vi "Xeryon Axis driver.vi"(4 "Config":T1, 5 "Stage index":u32) -> ()   [LabVIEW 2014]
uses:
  <vilib>/Utility/error.llb/DialogType.ctl
  Serial driver/Serial parameters.ctl
  Xeryon Axis command.ctl
  Xeryon status bits.ctl
  Axis Manager/Axis config.ctl
  Axis Manager/Axis enum.ctl
panel:
  out "Latched setpoint":dbl
  in  "Save":bool
  in  "Recover":bool
  in  "Reset encoder":bool
  in  "Apply settings file":bool
  in  "Settings file":path
  in  "Tab Control":enum32{"Status", "Graphs", "Feedback"}(tab)
  out "Within Tolerance":bool
  out "Statusbits":T3
  out "Actual position":dbl
  out "Serial number":i32
  out "Software number":i32
  out "Stage type":string
  out "Waveform Chart":T4(graph)
  out "Multicolumn Listbox":i32(listbox)
  in  "Continue":bool
  in  "Stop":bool
  in  "Go":bool
  in  "Desired speed":dbl=10.0
  in  "Desired position":dbl
  in  "Step size":dbl=1.0
  in  "Step +X":bool
  in  "Step -X":bool
  in  "Scan +X":bool
  in  "Scan -X":bool
  in  "Find index":bool
  in  "Reset":bool
  out "History :":i32(listbox)=-1
  out "Send feedback":bool
  # "Controls"
  # "In working units (°/mm)"
  # "In working units (°/mm)"
  # "Rotation :  deg/s  - Linear : mm/s"
  # "In working units"
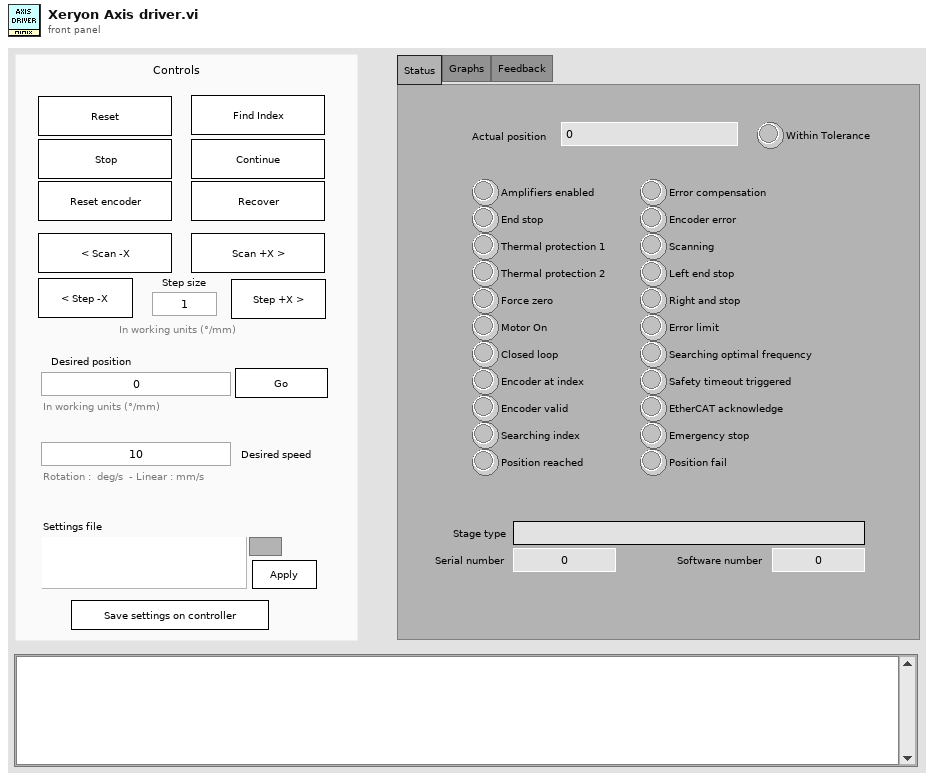
[diagram p1: front panel]
types:
  T1 = typedef "Axis config.ctl" = cluster{"Letter":string, "Stagetype":T2}
  T2 = typedef "Axis enum.ctl" = enum16{"XLA with 50 µm resolution", "XLA with 10 µm resolution", "XLA with 1250 nm resolution", "XLA with 312 nm resolution", "XLA with 78 nm resolution", "XLS with 1250 nm resolution", "XLS with 312 nm resolution", "XLS with 78nm resolution", "XLS with 5nm resolution", "XLS with 1 nm resolution", "XRT-A with 109 µrad resolution", "XRT-U-30 with 109 µrad resolution", "XRT-U-30 with 49 µrad resolution", "XRT-U-30 with 19 µrad resolution", "XRT-U-30 with 3 µrad resolution", "XRT-U-40 with 109 µrad resolution", "XRT-U 40 with 49 µrad resolution", "XRT-U-40 with 19 µrad resolution", "XRT-U-40 with 3 µrad resolution", "XRT-U-60 with 109 µrad resolution", "XRT-U-60 with 49 µrad resolution", "XRT-U-60 with 19 µrad resolution", "XRT-U-60 with 3 µrad resolution"}
  T3 = typedef "Xeryon status bits.ctl" = cluster{"Amplifiers enabled":bool, "End stop":bool, "Thermal protection 1":bool, "Thermal protection 2":bool, "Force zero":bool, "Motor On":bool, "Closed loop":bool, "Encoder at index":bool, "Encoder valid":bool, "Searching index":bool, "Position reached":bool, "Error compensation":bool, "Encoder error":bool, "Scanning":bool, "Left end stop":bool, "Right and stop":bool, "Error limit":bool, "Searching optimal frequency":bool, "Safety timeout triggered":bool, "EtherCAT acknowledge":bool, "Emergency stop":bool, "Position fail":bool}
  T4 = cluster{"Value out":dbl, "Latched setpoint":dbl, i16}
  T5 = enum16{"Position : From user units", "Position : To user units"}
  T6 = typedef "Xeryon Axis command.ctl" = cluster{"Command":enum16{"Reset", "Zero output", "Go home", "Find index", "Scan -X", "Scan +X", "Scan Stop", "Step -X", "Step +X", "Set DPOS", "Stop", "Continue", "Desired speed", "Apply settings file", "Exit", "Reset encoder", "Recover", "Save"}, "Data to send":string}
  T7 = enum16{"Init", "Set stage data", "Update position", "Get"}
  T8 = typedef "Serial parameters.ctl" = enum16{"Serial number", "Software number", "Type of stage", "Status", "Frequency", "Encoder position", "Desired position", "Info", "Phase correction", "Timestamp", "Proportional control factor", "Sync", "XRT1", "XRT3", "XRTA", "XLS1", "XLS3", "XLA1", "XLA3"}
  T9 = enum16{"Reset", "Zero output", "Go home", "Find index", "Scan -X", "Scan +X", "Scan Stop", "Step -X", "Step +X", "Set DPOS", "Stop", "Continue", "Desired speed", "Apply settings file", "Exit", "Reset encoder", "Recover", "Save"}
  T10 = cluster{"Parameters out":T8[], "Values out":i32[], "Stage type":string, "Stage letter":string}
  T11 = typedef "DialogType.ctl" = u16
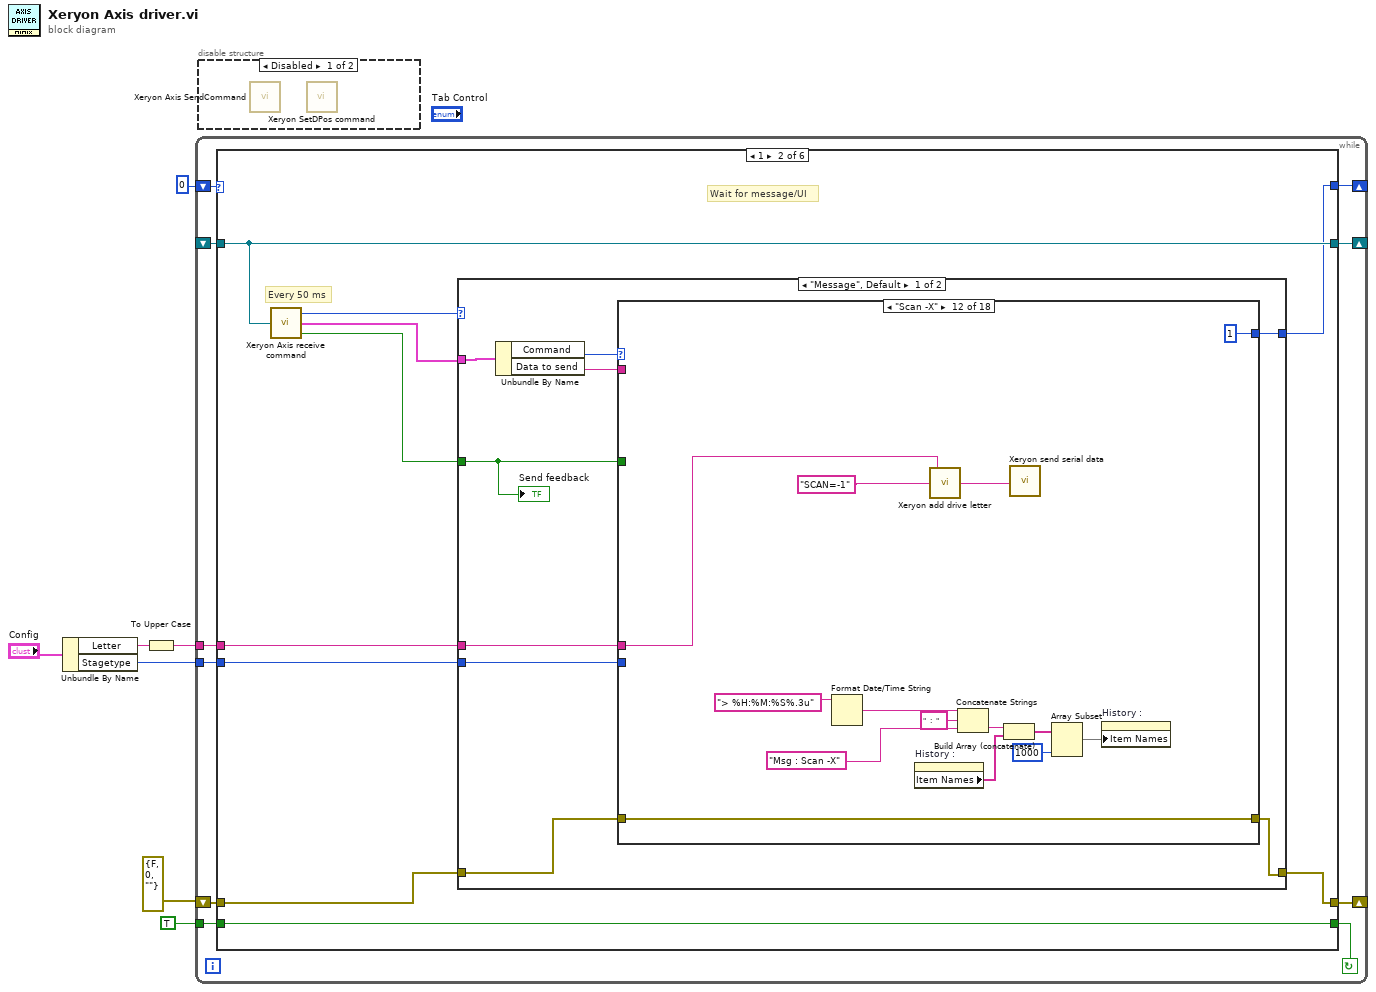
[diagram p0: block diagram]
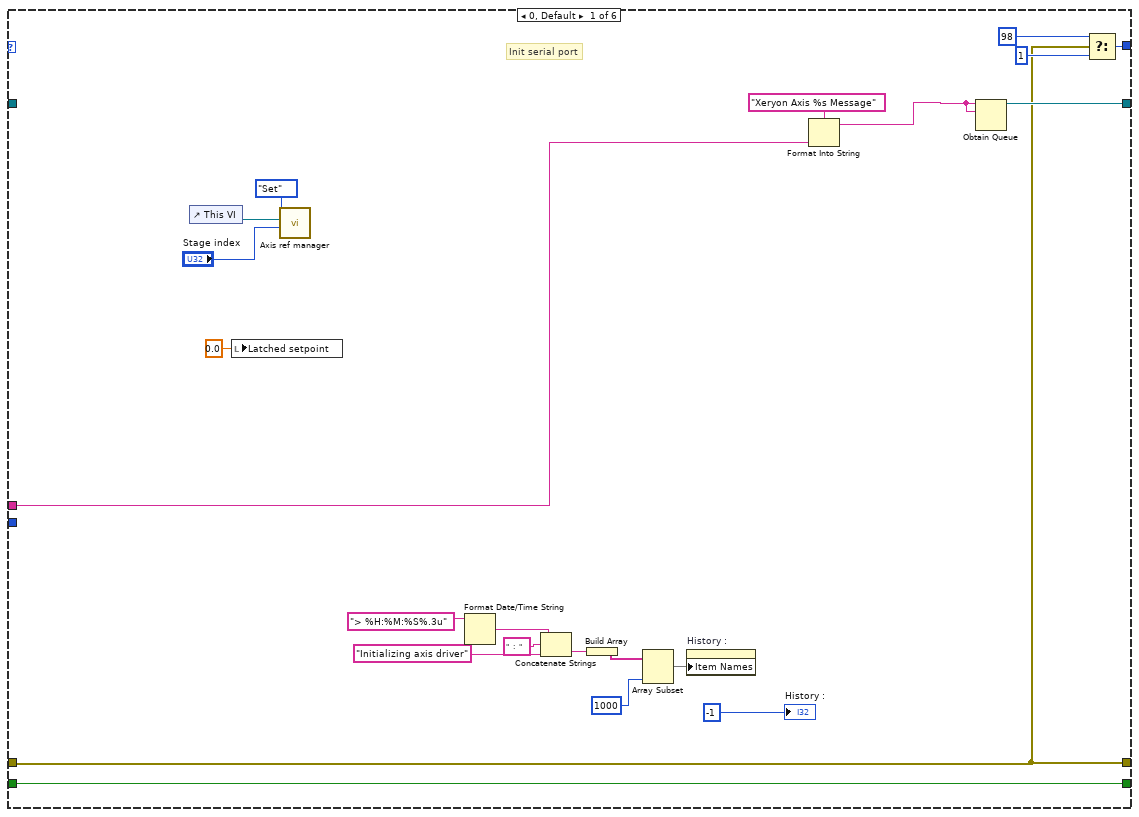
[diagram p3: hidden frame]
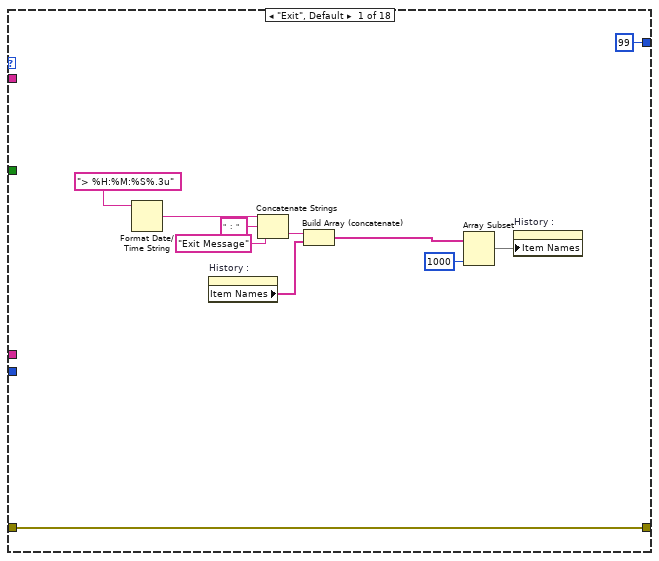
[diagram p4: hidden frame]
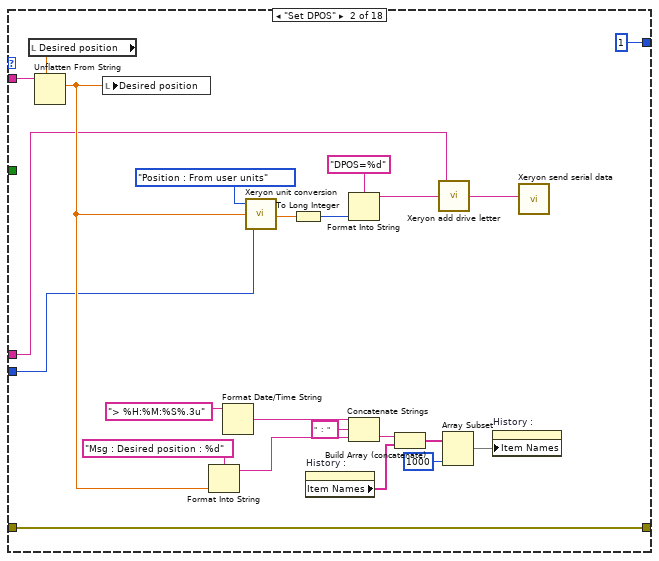
[diagram p5: hidden frame]
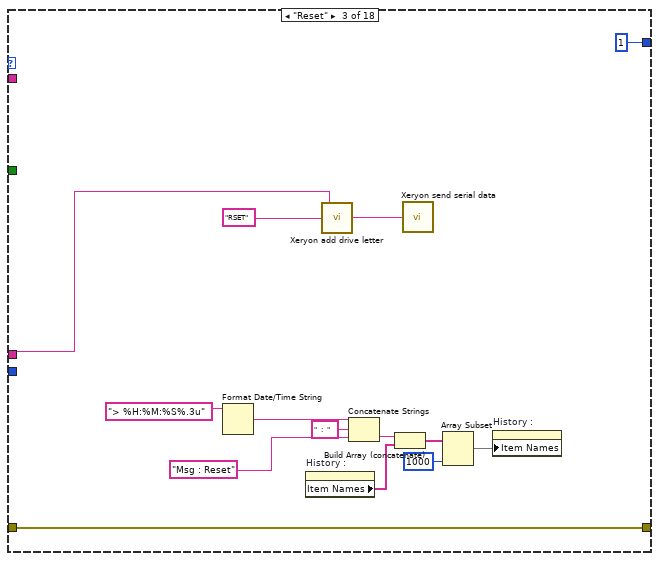
[diagram p6: hidden frame]
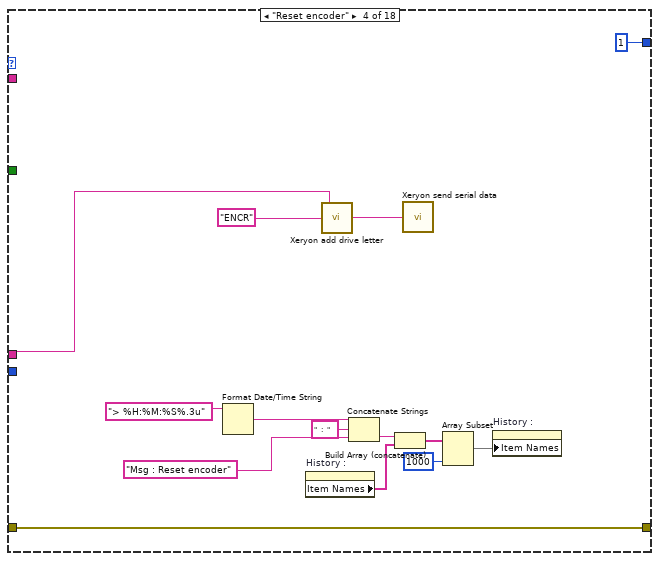
[diagram p7: hidden frame]
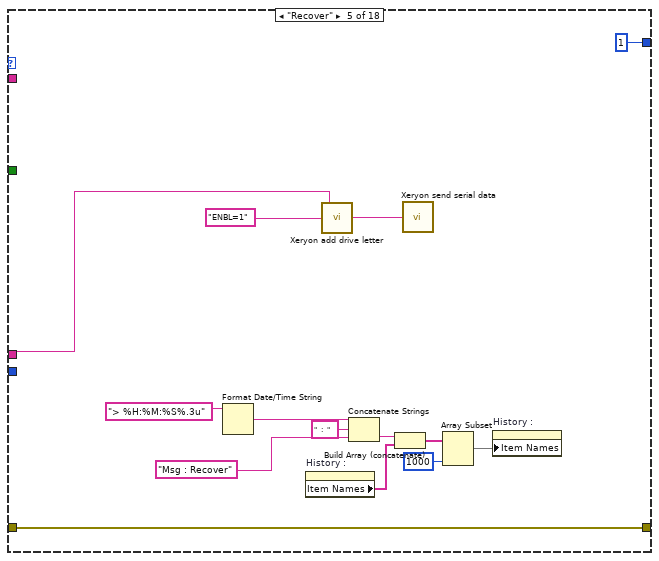
[diagram p8: hidden frame]
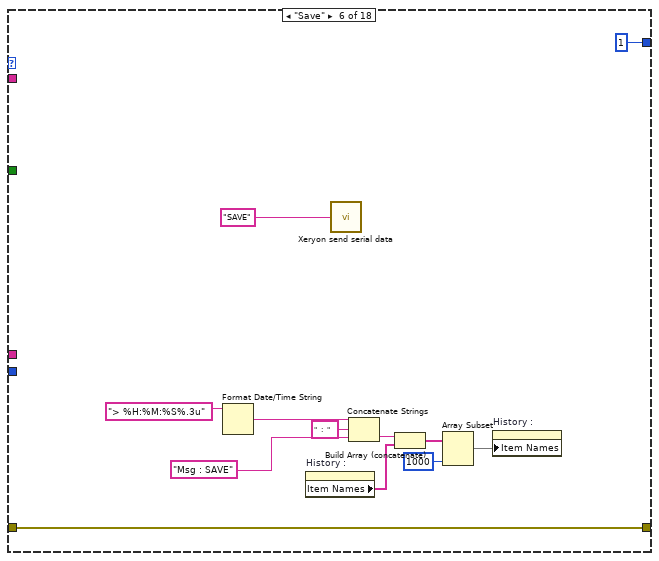
[diagram p9: hidden frame]
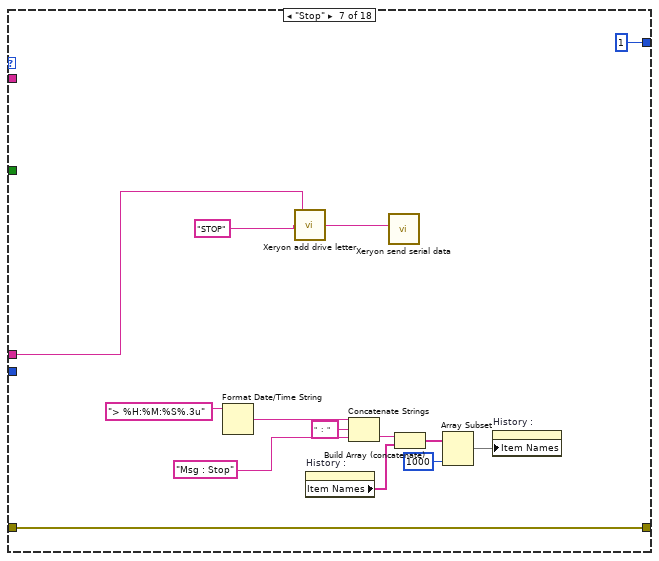
[diagram p10: hidden frame]
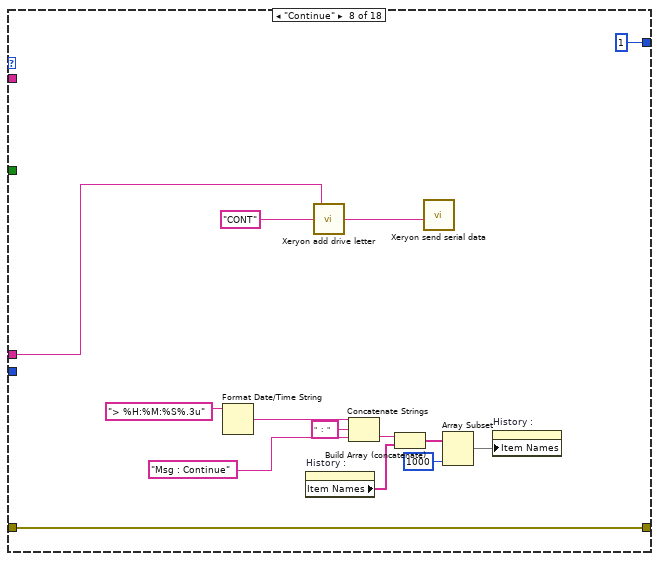
[diagram p11: hidden frame]
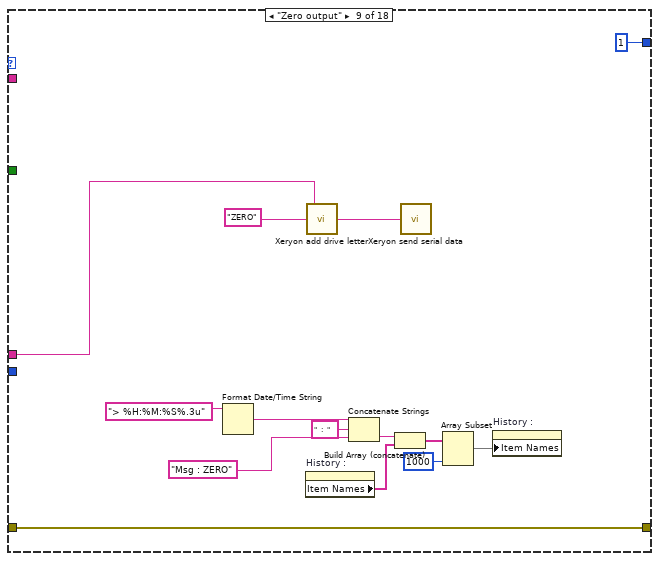
[diagram p12: hidden frame]
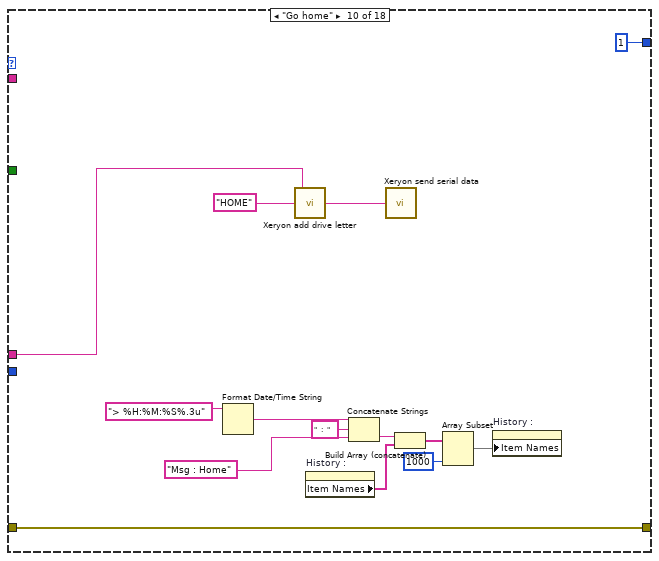
[diagram p13: hidden frame]
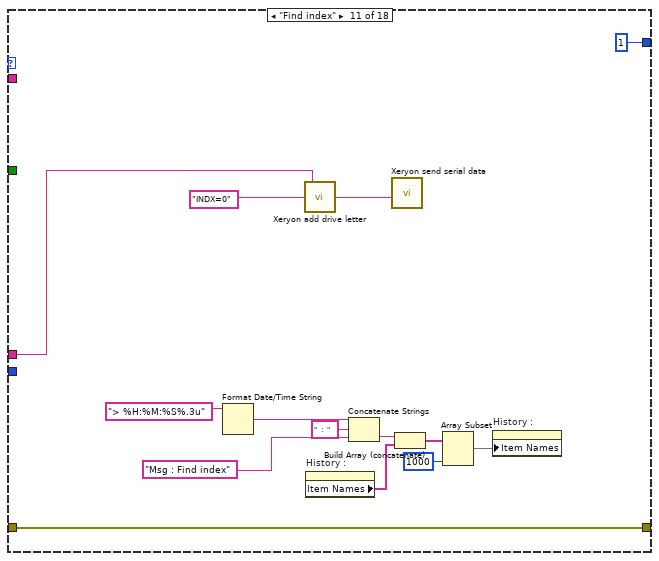
[diagram p14: hidden frame]
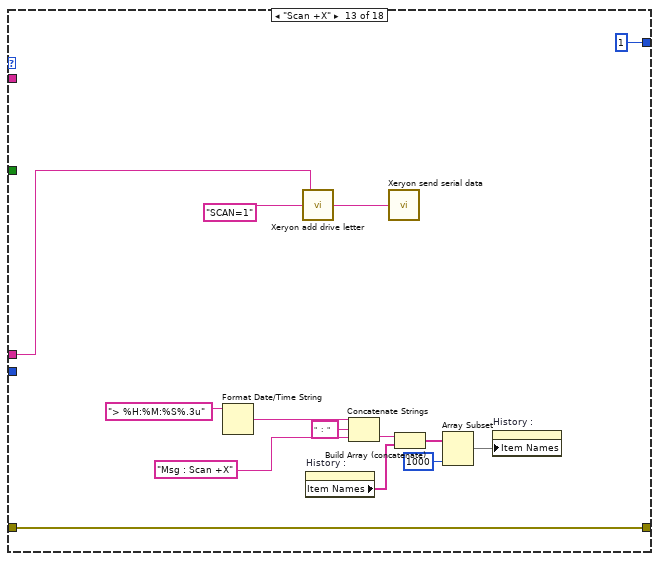
[diagram p15: hidden frame]
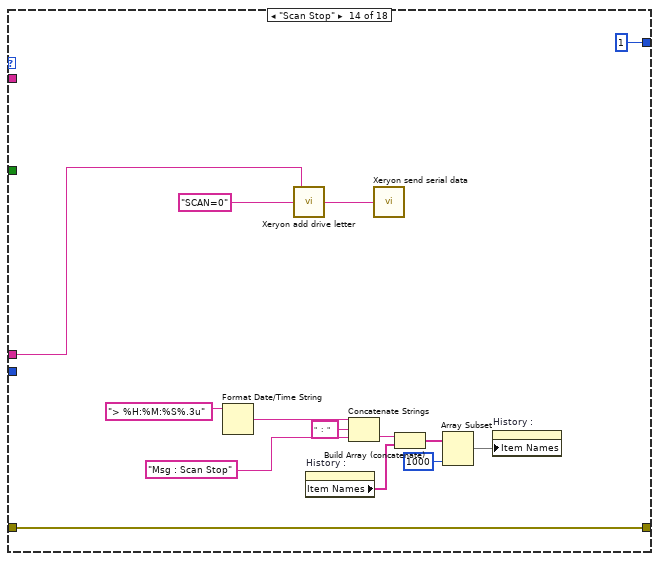
[diagram p16: hidden frame]
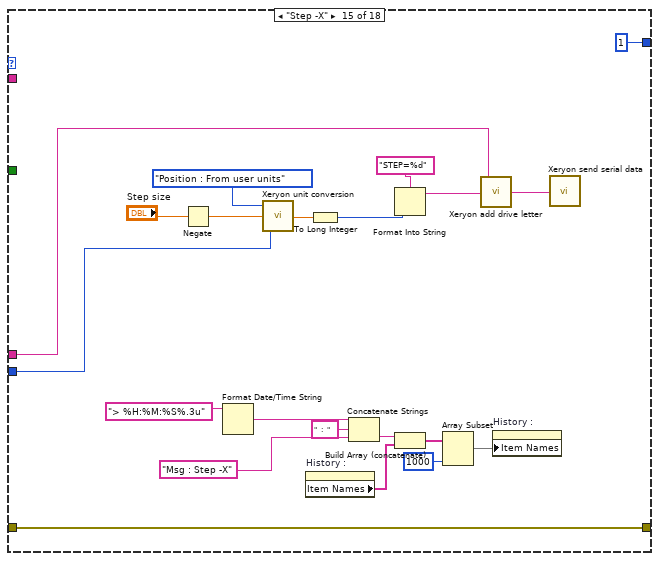
[diagram p17: hidden frame]
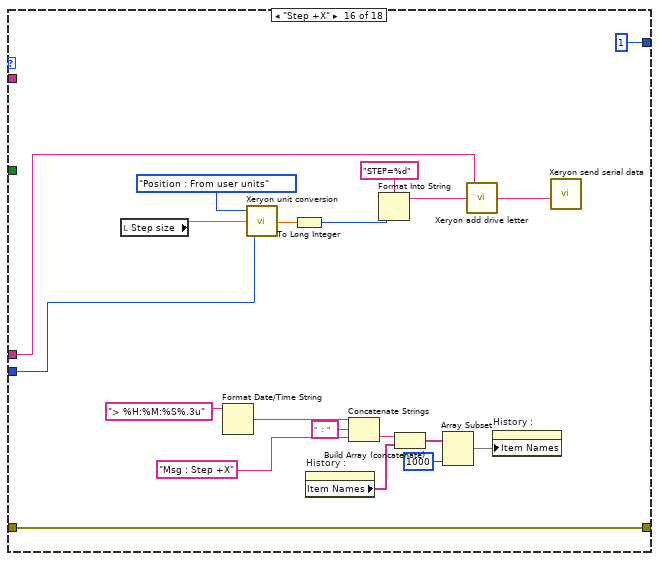
[diagram p18: hidden frame]
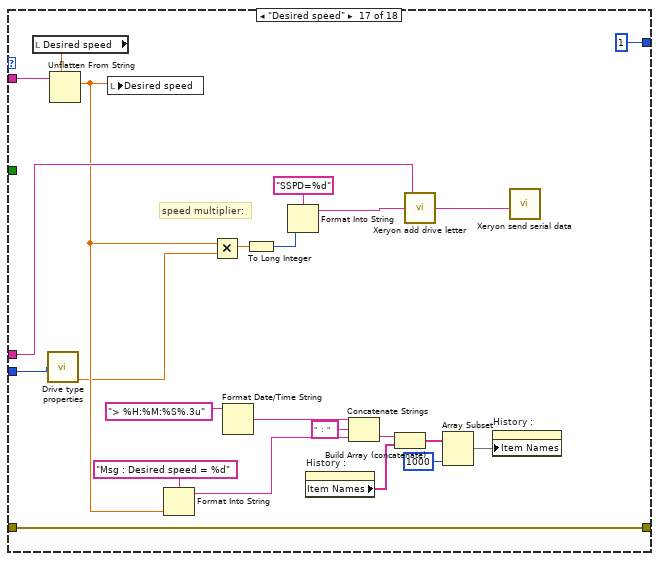
[diagram p19: hidden frame]
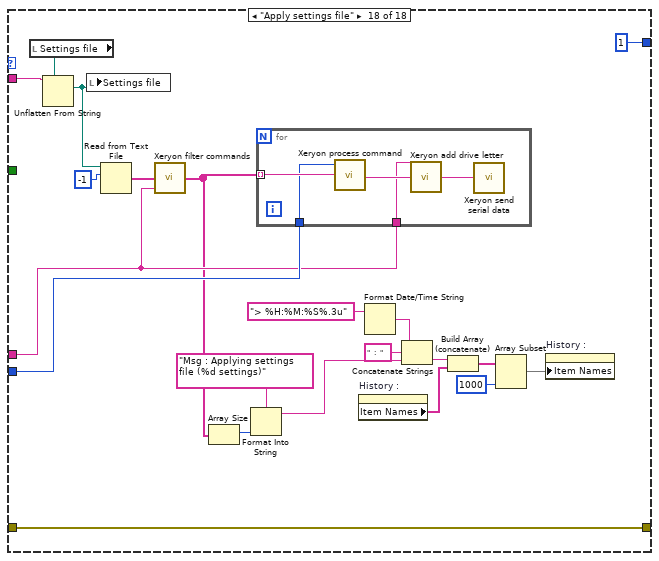
[diagram p20: hidden frame]
diagram:
  n1 = Unbundle By Name("Config") -> ("Letter"=w3:string, "Stagetype"=w2:T2)
  n2 = To Upper Case(1:w3) -> (0:w1:string)
  n3 = while {
    shift-right: [w12] -> _
    shift-left: 0 -> [w17]
    shift-right: [w13] -> _
    shift-left: errorcluster {"status"=FALSE, "code"=0, "source"=""} ("error in") -> [w16]
    tunnel: TRUE -> [w15]
    shift-right: [w11] -> _
    shift-left: _ -> [w10]
    tunnel: w1 -> [w9]
    tunnel: w2 -> [w8]
    stop <- w14 continue-if-true
    n4 = case shown="1" w17 {
      tunnel: w16 -> [w23 w44 w591 w602 w620 w638]
      tunnel: [w39 w49 w595 w603 w634 FALSE] -> w14
      tunnel: w15 -> [w39 w49 w595 w603 w634 _]
      tunnel: [w23 w43 w591 w602 errorcluster {"status"=FALSE, "code"=0, "source"=""} ("error in") w638] -> w13
      tunnel: [w38 w42 w592 1 ("t") 99 0] -> w12
      tunnel: [w35 w45 w596 w616 w633 w636] -> w11
      tunnel: w10 -> [_ w45 w596 w616 w633 w636]
      tunnel: w9 -> [w20 w41 w572 _ _ _]
      tunnel: w8 -> [_ w40 w575 _ _ _]
      frame 0, Default {
        # "Init serial port"
        n5 = control-ref of="This VI"() -> (w21:refnum<vi>)
        n6 = local write "Latched setpoint"(0.0 ("Latched setpoint")) -> ()
        n7 = call "Axis ref manager.vi"("Index/size in"="Stage index", "Ref in"=w21, "Mode"=enum16{"Init", "Set", "Get"}."Set") -> ()  [unwired: 4 in, 1 out]
        n8 = Format Date/Time String(time format string (%c)="> %H:%M:%S%.3u") -> (date/time string=w32:string)  [unwired: 2 out]
        n9 = Concatenate Strings(w32, "  :  " ("string"), "Initializing axis driver" ("string")) -> (w30:string)
        n10 = Build Array(w30) -> (w29:string[])
        n11 = Array Subset(array=w29, length=1000) -> (w26:string[])  [unwired: 1 in]
        n12 = property on="History :" class="LstBox (strict)"("Item Names"=w26) -> ()  [unwired: 2 in, 2 out]
        n13 = Format Into String(format string="Xeryon Axis %s Message" ("name (unnamed)"), w20) -> (resulting string=w24:string)  [unwired: 2 in, 1 out]
        n14 = Obtain Queue(name (unnamed)=w24, element data type=w24) -> (queue out=w35:refnum<queue>)  [unwired: 3 in, 2 out]
        n15 = Select(t=98, s=w23, f=1) -> (s? t:f=w38:i32)
        "History :" <- -1 ("History :")
      }
      frame 1 {
        # "Every 50 ms"
        # "Wait for message/UI"
        n16 = call "Xeryon Axis receive command.vi"("queue out"=w45) -> ("Type"=w48:enum16{"Message", "Timeout"}, "Serial Message"=w47:T6, "Send feedback"=w46:bool)
        n17 = case shown="\"Message\", Default" w48 {
          tunnel: w47 -> [w58 _]
          tunnel: [w55 w352] -> w42
          tunnel: [w53 w351] -> w43
          tunnel: w44 -> [w54 w351]
          tunnel: w46 -> [w52 _]
          tunnel: w41 -> [w51 w349]
          tunnel: w40 -> [w50 _]
          frame "Message", Default {
            n18 = Unbundle By Name(w58) -> ("Command"=w57:T9, "Data to send"=w56:string)
            n19 = case shown="\"Scan -X\"" w57 {
              tunnel: w56 -> [_ w82 _ _ _ _ _ _ _ _ _ _ _ _ _ _ w311 w329]
              tunnel: [99 1 1 1 1 1 1 1 1 1 1 1 1 1 1 1 1 1] -> w55
              tunnel: [w68 w91 w105 w119 w133 w145 w159 w173 w187 w201 w215 w229 w243 w257 w278 w298 w321 w342] -> w53
              tunnel: w54 -> [w68 w91 w105 w119 w133 w145 w159 w173 w187 w201 w215 w229 w243 w257 w278 w298 w321 w342]
              tunnel: w52 -> [_ _ _ _ _ _ _ _ _ _ _ _ _ _ _ _ _ _]
              tunnel: w51 -> [_ w70 w93 w107 w121 _ w147 w161 w175 w189 w203 w217 w231 w245 w259 w280 w305 w324]
              tunnel: w50 -> [_ w71 _ _ _ _ _ _ _ _ _ _ _ _ w260 w281 w301 w326]
              frame "Exit", Default {
                n20 = Format Date/Time String(time format string (%c)="> %H:%M:%S%.3u") -> (date/time string=w61:string)  [unwired: 2 out]
                n21 = property on="History :" class="LstBox (strict)"() -> ("Item Names"=w67:string[])  [unwired: 2 in, 2 out]
                n22 = Concatenate Strings(w61, "  :  " ("string"), "Exit Message" ("string")) -> (w64:string)
                n23 = Build Array (concatenate)(w64, w67) -> (w65:string[])
                n24 = Array Subset(array=w65, length=1000) -> (w59:string[])  [unwired: 1 in]
                n25 = property on="History :" class="LstBox (strict)"("Item Names"=w59) -> ()  [unwired: 2 in, 2 out]
              }
              frame "Set DPOS" {
                n26 = local read "Desired position"() -> (w81:dbl)
                n27 = Unflatten From String(type=w81, binary string=w82) -> (value=w76:dbl)  [unwired: 3 in, 2 out]
                n28 = local write "Desired position"(w76) -> ()
                n29 = Format Into String(format string="Msg : Desired position : %d" ("string"), w76) -> (resulting string=w79:string)  [unwired: 2 in, 1 out]
                n30 = Format Date/Time String(time format string (%c)="> %H:%M:%S%.3u") -> (date/time string=w85:string)  [unwired: 2 out]
                n31 = call "Xeryon unit conversion.vi"("Type"=w71, "Value in"=w76, "Mode"=T5."Position : From user units") -> ("Value out"=w75:dbl)  [unwired: 2 in]
                n32 = To Long Integer(number=w75) -> (32bit integer=w74:i32)
                n33 = property on="History :" class="LstBox (strict)"() -> ("Item Names"=w90:string[])  [unwired: 2 in, 2 out]
                n34 = Format Into String(format string="DPOS=%d" ("Data to send"), w74) -> (resulting string=w73:string)  [unwired: 2 in, 1 out]
                n35 = Concatenate Strings(w85, "  :  " ("string"), w79) -> (w87:string)
                n36 = Build Array (concatenate)(w87, w90) -> (w88:string[])
                n37 = call "Xeryon add drive letter.vi"("String in"=w73, "Drive letter"=w70) -> ("String out"=w72:string)  [unwired: 3 in]
                n38 = Array Subset(array=w88, length=1000) -> (w83:string[])  [unwired: 1 in]
                n39 = property on="History :" class="LstBox (strict)"("Item Names"=w83) -> ()  [unwired: 2 in, 2 out]
                n40 = call "Xeryon send serial data.vi"("Data to send"=w72) -> ()  [unwired: 5 in]
              }
              frame "Reset" {
                n41 = Format Date/Time String(time format string (%c)="> %H:%M:%S%.3u") -> (date/time string=w99:string)  [unwired: 2 out]
                n42 = property on="History :" class="LstBox (strict)"() -> ("Item Names"=w104:string[])  [unwired: 2 in, 2 out]
                n43 = call "Xeryon add drive letter.vi"("String in"="RSET" ("Data to send"), "Drive letter"=w93) -> ("String out"=w94:string)  [unwired: 3 in]
                n44 = Concatenate Strings(w99, "  :  " ("string"), "Msg : Reset" ("string")) -> (w101:string)
                n45 = Build Array (concatenate)(w101, w104) -> (w102:string[])
                n46 = call "Xeryon send serial data.vi"("Data to send"=w94) -> ()  [unwired: 5 in]
                n47 = Array Subset(array=w102, length=1000) -> (w97:string[])  [unwired: 1 in]
                n48 = property on="History :" class="LstBox (strict)"("Item Names"=w97) -> ()  [unwired: 2 in, 2 out]
              }
              frame "Reset encoder" {
                n49 = Format Date/Time String(time format string (%c)="> %H:%M:%S%.3u") -> (date/time string=w113:string)  [unwired: 2 out]
                n50 = property on="History :" class="LstBox (strict)"() -> ("Item Names"=w118:string[])  [unwired: 2 in, 2 out]
                n51 = call "Xeryon add drive letter.vi"("String in"="ENCR" ("Data to send"), "Drive letter"=w107) -> ("String out"=w108:string)  [unwired: 3 in]
                n52 = Concatenate Strings(w113, "  :  " ("string"), "Msg : Reset encoder" ("string")) -> (w115:string)
                n53 = Build Array (concatenate)(w115, w118) -> (w116:string[])
                n54 = call "Xeryon send serial data.vi"("Data to send"=w108) -> ()  [unwired: 5 in]
                n55 = Array Subset(array=w116, length=1000) -> (w111:string[])  [unwired: 1 in]
                n56 = property on="History :" class="LstBox (strict)"("Item Names"=w111) -> ()  [unwired: 2 in, 2 out]
              }
              frame "Recover" {
                n57 = Format Date/Time String(time format string (%c)="> %H:%M:%S%.3u") -> (date/time string=w127:string)  [unwired: 2 out]
                n58 = property on="History :" class="LstBox (strict)"() -> ("Item Names"=w132:string[])  [unwired: 2 in, 2 out]
                n59 = call "Xeryon add drive letter.vi"("String in"="ENBL=1" ("Data to send"), "Drive letter"=w121) -> ("String out"=w122:string)  [unwired: 3 in]
                n60 = Concatenate Strings(w127, "  :  " ("string"), "Msg : Recover" ("string")) -> (w129:string)
                n61 = Build Array (concatenate)(w129, w132) -> (w130:string[])
                n62 = call "Xeryon send serial data.vi"("Data to send"=w122) -> ()  [unwired: 5 in]
                n63 = Array Subset(array=w130, length=1000) -> (w125:string[])  [unwired: 1 in]
                n64 = property on="History :" class="LstBox (strict)"("Item Names"=w125) -> ()  [unwired: 2 in, 2 out]
              }
              frame "Save" {
                n65 = Format Date/Time String(time format string (%c)="> %H:%M:%S%.3u") -> (date/time string=w139:string)  [unwired: 2 out]
                n66 = property on="History :" class="LstBox (strict)"() -> ("Item Names"=w144:string[])  [unwired: 2 in, 2 out]
                n67 = call "Xeryon send serial data.vi"("Data to send"="SAVE") -> ()  [unwired: 5 in]
                n68 = Concatenate Strings(w139, "  :  " ("string"), "Msg : SAVE" ("string")) -> (w141:string)
                n69 = Build Array (concatenate)(w141, w144) -> (w142:string[])
                n70 = Array Subset(array=w142, length=1000) -> (w137:string[])  [unwired: 1 in]
                n71 = property on="History :" class="LstBox (strict)"("Item Names"=w137) -> ()  [unwired: 2 in, 2 out]
              }
              frame "Stop" {
                n72 = Format Date/Time String(time format string (%c)="> %H:%M:%S%.3u") -> (date/time string=w153:string)  [unwired: 2 out]
                n73 = call "Xeryon add drive letter.vi"("String in"="STOP" ("Data to send"), "Drive letter"=w147) -> ("String out"=w148:string)  [unwired: 3 in]
                n74 = property on="History :" class="LstBox (strict)"() -> ("Item Names"=w158:string[])  [unwired: 2 in, 2 out]
                n75 = Concatenate Strings(w153, "  :  " ("string"), "Msg : Stop" ("string")) -> (w155:string)
                n76 = call "Xeryon send serial data.vi"("Data to send"=w148) -> ()  [unwired: 5 in]
                n77 = Build Array (concatenate)(w155, w158) -> (w156:string[])
                n78 = Array Subset(array=w156, length=1000) -> (w151:string[])  [unwired: 1 in]
                n79 = property on="History :" class="LstBox (strict)"("Item Names"=w151) -> ()  [unwired: 2 in, 2 out]
              }
              frame "Continue" {
                n80 = Format Date/Time String(time format string (%c)="> %H:%M:%S%.3u") -> (date/time string=w167:string)  [unwired: 2 out]
                n81 = property on="History :" class="LstBox (strict)"() -> ("Item Names"=w172:string[])  [unwired: 2 in, 2 out]
                n82 = call "Xeryon add drive letter.vi"("String in"="CONT" ("Data to send"), "Drive letter"=w161) -> ("String out"=w162:string)  [unwired: 3 in]
                n83 = Concatenate Strings(w167, "  :  " ("string"), "Msg : Continue" ("string")) -> (w169:string)
                n84 = Build Array (concatenate)(w169, w172) -> (w170:string[])
                n85 = call "Xeryon send serial data.vi"("Data to send"=w162) -> ()  [unwired: 5 in]
                n86 = Array Subset(array=w170, length=1000) -> (w165:string[])  [unwired: 1 in]
                n87 = property on="History :" class="LstBox (strict)"("Item Names"=w165) -> ()  [unwired: 2 in, 2 out]
              }
              frame "Zero output" {
                n88 = Format Date/Time String(time format string (%c)="> %H:%M:%S%.3u") -> (date/time string=w181:string)  [unwired: 2 out]
                n89 = property on="History :" class="LstBox (strict)"() -> ("Item Names"=w186:string[])  [unwired: 2 in, 2 out]
                n90 = call "Xeryon add drive letter.vi"("String in"="ZERO" ("Data to send"), "Drive letter"=w175) -> ("String out"=w176:string)  [unwired: 3 in]
                n91 = Concatenate Strings(w181, "  :  " ("string"), "Msg : ZERO" ("string")) -> (w183:string)
                n92 = Build Array (concatenate)(w183, w186) -> (w184:string[])
                n93 = call "Xeryon send serial data.vi"("Data to send"=w176) -> ()  [unwired: 5 in]
                n94 = Array Subset(array=w184, length=1000) -> (w179:string[])  [unwired: 1 in]
                n95 = property on="History :" class="LstBox (strict)"("Item Names"=w179) -> ()  [unwired: 2 in, 2 out]
              }
              frame "Go home" {
                n96 = Format Date/Time String(time format string (%c)="> %H:%M:%S%.3u") -> (date/time string=w195:string)  [unwired: 2 out]
                n97 = call "Xeryon add drive letter.vi"("String in"="HOME" ("Data to send"), "Drive letter"=w189) -> ("String out"=w190:string)  [unwired: 3 in]
                n98 = property on="History :" class="LstBox (strict)"() -> ("Item Names"=w200:string[])  [unwired: 2 in, 2 out]
                n99 = Concatenate Strings(w195, "  :  " ("string"), "Msg : Home" ("string")) -> (w197:string)
                n100 = call "Xeryon send serial data.vi"("Data to send"=w190) -> ()  [unwired: 5 in]
                n101 = Build Array (concatenate)(w197, w200) -> (w198:string[])
                n102 = Array Subset(array=w198, length=1000) -> (w193:string[])  [unwired: 1 in]
                n103 = property on="History :" class="LstBox (strict)"("Item Names"=w193) -> ()  [unwired: 2 in, 2 out]
              }
              frame "Find index" {
                n104 = Format Date/Time String(time format string (%c)="> %H:%M:%S%.3u") -> (date/time string=w209:string)  [unwired: 2 out]
                n105 = call "Xeryon add drive letter.vi"("String in"="INDX=0" ("Data to send"), "Drive letter"=w203) -> ("String out"=w204:string)  [unwired: 3 in]
                n106 = property on="History :" class="LstBox (strict)"() -> ("Item Names"=w214:string[])  [unwired: 2 in, 2 out]
                n107 = Concatenate Strings(w209, "  :  " ("string"), "Msg : Find index" ("string")) -> (w211:string)
                n108 = call "Xeryon send serial data.vi"("Data to send"=w204) -> ()  [unwired: 5 in]
                n109 = Build Array (concatenate)(w211, w214) -> (w212:string[])
                n110 = Array Subset(array=w212, length=1000) -> (w207:string[])  [unwired: 1 in]
                n111 = property on="History :" class="LstBox (strict)"("Item Names"=w207) -> ()  [unwired: 2 in, 2 out]
              }
              frame "Scan -X" {
                n112 = Format Date/Time String(time format string (%c)="> %H:%M:%S%.3u") -> (date/time string=w223:string)  [unwired: 2 out]
                n113 = property on="History :" class="LstBox (strict)"() -> ("Item Names"=w228:string[])  [unwired: 2 in, 2 out]
                n114 = call "Xeryon add drive letter.vi"("String in"="SCAN=-1" ("Data to send"), "Drive letter"=w217) -> ("String out"=w218:string)  [unwired: 3 in]
                n115 = Concatenate Strings(w223, "  :  " ("string"), "Msg : Scan -X" ("string")) -> (w225:string)
                n116 = Build Array (concatenate)(w225, w228) -> (w226:string[])
                n117 = call "Xeryon send serial data.vi"("Data to send"=w218) -> ()  [unwired: 5 in]
                n118 = Array Subset(array=w226, length=1000) -> (w221:string[])  [unwired: 1 in]
                n119 = property on="History :" class="LstBox (strict)"("Item Names"=w221) -> ()  [unwired: 2 in, 2 out]
              }
              frame "Scan +X" {
                n120 = Format Date/Time String(time format string (%c)="> %H:%M:%S%.3u") -> (date/time string=w237:string)  [unwired: 2 out]
                n121 = call "Xeryon add drive letter.vi"("String in"="SCAN=1" ("Data to send"), "Drive letter"=w231) -> ("String out"=w232:string)  [unwired: 3 in]
                n122 = property on="History :" class="LstBox (strict)"() -> ("Item Names"=w242:string[])  [unwired: 2 in, 2 out]
                n123 = Concatenate Strings(w237, "  :  " ("string"), "Msg : Scan +X" ("string")) -> (w239:string)
                n124 = call "Xeryon send serial data.vi"("Data to send"=w232) -> ()  [unwired: 5 in]
                n125 = Build Array (concatenate)(w239, w242) -> (w240:string[])
                n126 = Array Subset(array=w240, length=1000) -> (w235:string[])  [unwired: 1 in]
                n127 = property on="History :" class="LstBox (strict)"("Item Names"=w235) -> ()  [unwired: 2 in, 2 out]
              }
              frame "Scan Stop" {
                n128 = Format Date/Time String(time format string (%c)="> %H:%M:%S%.3u") -> (date/time string=w251:string)  [unwired: 2 out]
                n129 = call "Xeryon add drive letter.vi"("String in"="SCAN=0" ("Data to send"), "Drive letter"=w245) -> ("String out"=w246:string)  [unwired: 3 in]
                n130 = property on="History :" class="LstBox (strict)"() -> ("Item Names"=w256:string[])  [unwired: 2 in, 2 out]
                n131 = Concatenate Strings(w251, "  :  " ("string"), "Msg : Scan Stop" ("string")) -> (w253:string)
                n132 = call "Xeryon send serial data.vi"("Data to send"=w246) -> ()  [unwired: 5 in]
                n133 = Build Array (concatenate)(w253, w256) -> (w254:string[])
                n134 = Array Subset(array=w254, length=1000) -> (w249:string[])  [unwired: 1 in]
                n135 = property on="History :" class="LstBox (strict)"("Item Names"=w249) -> ()  [unwired: 2 in, 2 out]
              }
              frame "Step -X" {
                n136 = Negate(x="Step size") -> (-x=w264:dbl)
                n137 = Format Date/Time String(time format string (%c)="> %H:%M:%S%.3u") -> (date/time string=w272:string)  [unwired: 2 out]
                n138 = call "Xeryon unit conversion.vi"("Type"=w260, "Value in"=w264, "Mode"=T5."Position : From user units") -> ("Value out"=w266:dbl)  [unwired: 2 in]
                n139 = property on="History :" class="LstBox (strict)"() -> ("Item Names"=w277:string[])  [unwired: 2 in, 2 out]
                n140 = To Long Integer(number=w266) -> (32bit integer=w263:i32)
                n141 = Concatenate Strings(w272, "  :  " ("string"), "Msg : Step -X" ("string")) -> (w274:string)
                n142 = Format Into String(format string="STEP=%d" ("Data to send"), w263) -> (resulting string=w262:string)  [unwired: 2 in, 1 out]
                n143 = Build Array (concatenate)(w274, w277) -> (w275:string[])
                n144 = Array Subset(array=w275, length=1000) -> (w270:string[])  [unwired: 1 in]
                n145 = call "Xeryon add drive letter.vi"("String in"=w262, "Drive letter"=w259) -> ("String out"=w261:string)  [unwired: 3 in]
                n146 = property on="History :" class="LstBox (strict)"("Item Names"=w270) -> ()  [unwired: 2 in, 2 out]
                n147 = call "Xeryon send serial data.vi"("Data to send"=w261) -> ()  [unwired: 5 in]
              }
              frame "Step +X" {
                n148 = local read "Step size"() -> (w284:dbl)
                n149 = Format Date/Time String(time format string (%c)="> %H:%M:%S%.3u") -> (date/time string=w292:string)  [unwired: 2 out]
                n150 = call "Xeryon unit conversion.vi"("Type"=w281, "Value in"=w284, "Mode"=T5."Position : From user units") -> ("Value out"=w288:dbl)  [unwired: 2 in]
                n151 = To Long Integer(number=w288) -> (32bit integer=w287:i32)
                n152 = property on="History :" class="LstBox (strict)"() -> ("Item Names"=w297:string[])  [unwired: 2 in, 2 out]
                n153 = Concatenate Strings(w292, "  :  " ("string"), "Msg : Step +X" ("string")) -> (w294:string)
                n154 = Format Into String(format string="STEP=%d" ("Data to send"), w287) -> (resulting string=w283:string)  [unwired: 2 in, 1 out]
                n155 = Build Array (concatenate)(w294, w297) -> (w295:string[])
                n156 = Array Subset(array=w295, length=1000) -> (w290:string[])  [unwired: 1 in]
                n157 = call "Xeryon add drive letter.vi"("String in"=w283, "Drive letter"=w280) -> ("String out"=w282:string)  [unwired: 3 in]
                n158 = property on="History :" class="LstBox (strict)"("Item Names"=w290) -> ()  [unwired: 2 in, 2 out]
                n159 = call "Xeryon send serial data.vi"("Data to send"=w282) -> ()  [unwired: 5 in]
              }
              frame "Desired speed" {
                # "speed multiplier:"
                n160 = local read "Desired speed"() -> (w310:dbl)
                n161 = call "Drive type properties.vi"("Type"=w301) -> ("Speed multiplier"=w300:dbl)  [unwired: 2 in, 3 out]
                n162 = Unflatten From String(type=w310, binary string=w311) -> (value=w304:dbl)  [unwired: 3 in, 2 out]
                n163 = local write "Desired speed"(w304) -> ()
                n164 = Format Into String(format string="Msg : Desired speed = %d" ("string"), w304) -> (resulting string=w308:string)  [unwired: 2 in, 1 out]
                n165 = Multiply(x=w304, y=w300) -> (x*y=w303:dbl)
                n166 = Format Date/Time String(time format string (%c)="> %H:%M:%S%.3u") -> (date/time string=w315:string)  [unwired: 2 out]
                n167 = To Long Integer(number=w303) -> (32bit integer=w302:i32)
                n168 = Format Into String(format string="SSPD=%d" ("Data to send"), w302) -> (resulting string=w307:string)  [unwired: 2 in, 1 out]
                n169 = property on="History :" class="LstBox (strict)"() -> ("Item Names"=w320:string[])  [unwired: 2 in, 2 out]
                n170 = Concatenate Strings(w315, "  :  " ("string"), w308) -> (w317:string)
                n171 = Build Array (concatenate)(w317, w320) -> (w318:string[])
                n172 = call "Xeryon add drive letter.vi"("String in"=w307, "Drive letter"=w305) -> ("String out"=w306:string)  [unwired: 3 in]
                n173 = Array Subset(array=w318, length=1000) -> (w313:string[])  [unwired: 1 in]
                n174 = property on="History :" class="LstBox (strict)"("Item Names"=w313) -> ()  [unwired: 2 in, 2 out]
                n175 = call "Xeryon send serial data.vi"("Data to send"=w306) -> ()  [unwired: 5 in]
              }
              frame "Apply settings file" {
                n176 = local read "Settings file"() -> (w328:path)
                n177 = Unflatten From String(type=w328, binary string=w329) -> (value=w327:path)  [unwired: 3 in, 2 out]
                n178 = local write "Settings file"(w327) -> ()
                n179 = Read from Text File(file (use dialog)=w327, count=-1) -> (text=w325:string[])  [unwired: 2 in, 3 out]
                n180 = call "Xeryon filter commands.vi"("Letter in"=w324, "Commands in"=w325) -> ("Commands out"=w323:string[])  [unwired: 3 in]
                n181 = Array Size(array=w323) -> (size(s)=w335:i32)
                n182 = Format Into String(format string="Msg : Applying settings file (%d settings)" ("string"), w335) -> (resulting string=w336:string)  [unwired: 2 in, 1 out]
                n183 = for {
                  tunnel: w323 -> [w348] mode=indexing
                  tunnel: w326 -> [w345]
                  tunnel: w324 -> [w344]
                  n184 = call "Xeryon process command.vi"("Command in"=w348, "Type"=w345) -> ("Command out"=w347:string)  [unwired: 3 in]
                  n185 = call "Xeryon add drive letter.vi"("String in"=w347, "Drive letter"=w344) -> ("String out"=w346:string)  [unwired: 3 in]
                  n186 = call "Xeryon send serial data.vi"("Data to send"=w346) -> ()  [unwired: 5 in]
                }
                n187 = property on="History :" class="LstBox (strict)"() -> ("Item Names"=w341:string[])  [unwired: 2 in, 2 out]
                n188 = Format Date/Time String(time format string (%c)="> %H:%M:%S%.3u") -> (date/time string=w338:string)  [unwired: 2 out]
                n189 = Concatenate Strings(w338, "  :  " ("string"), w336) -> (w339:string)
                n190 = Build Array (concatenate)(w339, w341) -> (w340:string[])
                n191 = Array Subset(array=w340, length=1000) -> (w337:string[])  [unwired: 1 in]
                n192 = property on="History :" class="LstBox (strict)"("Item Names"=w337) -> ()  [unwired: 2 in, 2 out]
              }
            }
            "Send feedback" <- w52
          }
          frame "Timeout" {
            n193 = event shown="[10] \"Go\": Value Change" {
              selector: _ -> [_ _ _ _ _ _ _ _ _ _ _ _ _ _ _]
              dyn-events: _ -> [_ _ _ _ _ _ _ _ _ _ _ _ _ _ _]
              timeout: 0 -> [_ _ _ _ _ _ _ _ _ _ _ _ _ _ _]
              tunnel: [2 1 1 1 1 1 1 1 1 1 1 1 1 1 1] -> w352
              tunnel: w349 -> [_ w355 w370 w385 w398 w410 w423 w436 w450 w462 w478 w493 w511 w530 w543]
              event Timeout {
                n194 = event-data() -> ()  [unwired: 3 out]
              }
              event "Reset": Value Change {
                n195 = event-data() -> ()  [unwired: 7 out]
                n196 = Format Date/Time String(time format string (%c)="> %H:%M:%S%.3u") -> (date/time string=w365:string)  [unwired: 2 out]
                n197 = property on="History :" class="LstBox (strict)"() -> ("Item Names"=w362:string[])  [unwired: 2 in, 2 out]
                n198 = Concatenate Strings(w365, "  :  " ("string"), "GUI : Reset axis" ("string")) -> (w364:string)
                n199 = Build Array (concatenate)(w364, w362) -> (w363:string[])
                n200 = Array Subset(array=w363, length=1000) -> (w361:string[])  [unwired: 1 in]
                n201 = call "Xeryon Axis SendCommand.vi"("Feedback?"=FALSE, "Stage"=w355, "Axis Command"=T6 {"Command"=enum."Reset", "Data to send"=""} ("Axis Message")) -> ()  [unwired: 3 in, 1 out]
                n202 = property on="History :" class="LstBox (strict)"("Item Names"=w361) -> ()  [unwired: 2 in, 2 out]
              }
              event "Save": Value Change {
                n203 = event-data() -> ()  [unwired: 7 out]
                n204 = Two Button Dialog(message="Are you sure you want to save the current parameters in the controllers firmware?", 2:"Save" ("T button name (\"OK\")")) -> (T button?=w367:bool)  [unwired: 1 in]
                n205 = case shown="True" w367 {
                  tunnel: w370 -> [_ w373]
                  frame False {
                  }
                  frame True {
                    n206 = Format Date/Time String(time format string (%c)="> %H:%M:%S%.3u") -> (date/time string=w383:string)  [unwired: 2 out]
                    n207 = property on="History :" class="LstBox (strict)"() -> ("Item Names"=w380:string[])  [unwired: 2 in, 2 out]
                    n208 = call "Xeryon Axis SendCommand.vi"("Feedback?"=FALSE, "Stage"=w373, "Axis Command"=T6 {"Command"=enum."Save", "Data to send"=""} ("Axis Message")) -> ()  [unwired: 3 in, 1 out]
                    n209 = Concatenate Strings(w383, "  :  " ("string"), "GUI : Reset axis" ("string")) -> (w382:string)
                    n210 = Build Array (concatenate)(w382, w380) -> (w381:string[])
                    n211 = Array Subset(array=w381, length=1000) -> (w379:string[])  [unwired: 1 in]
                    n212 = property on="History :" class="LstBox (strict)"("Item Names"=w379) -> ()  [unwired: 2 in, 2 out]
                  }
                }
              }
              event "Reset encoder": Value Change {
                n213 = event-data() -> ()  [unwired: 7 out]
                n214 = Format Date/Time String(time format string (%c)="> %H:%M:%S%.3u") -> (date/time string=w395:string)  [unwired: 2 out]
                n215 = property on="History :" class="LstBox (strict)"() -> ("Item Names"=w392:string[])  [unwired: 2 in, 2 out]
                n216 = Concatenate Strings(w395, "  :  " ("string"), "GUI : Reset encoder" ("string")) -> (w394:string)
                n217 = Build Array (concatenate)(w394, w392) -> (w393:string[])
                n218 = Array Subset(array=w393, length=1000) -> (w391:string[])  [unwired: 1 in]
                n219 = call "Xeryon Axis SendCommand.vi"("Feedback?"=FALSE, "Stage"=w385, "Axis Command"=T6 {"Command"=enum."Reset encoder", "Data to send"=""} ("Axis Message")) -> ()  [unwired: 3 in, 1 out]
                n220 = property on="History :" class="LstBox (strict)"("Item Names"=w391) -> ()  [unwired: 2 in, 2 out]
              }
              event "Recover": Value Change {
                n221 = event-data() -> ()  [unwired: 7 out]
                n222 = Format Date/Time String(time format string (%c)="> %H:%M:%S%.3u") -> (date/time string=w408:string)  [unwired: 2 out]
                n223 = property on="History :" class="LstBox (strict)"() -> ("Item Names"=w405:string[])  [unwired: 2 in, 2 out]
                n224 = Concatenate Strings(w408, "  :  " ("string"), "GUI : Recover" ("string")) -> (w407:string)
                n225 = Build Array (concatenate)(w407, w405) -> (w406:string[])
                n226 = Array Subset(array=w406, length=1000) -> (w404:string[])  [unwired: 1 in]
                n227 = call "Xeryon Axis SendCommand.vi"("Feedback?"=FALSE, "Stage"=w398, "Axis Command"=T6 {"Command"=enum."Recover", "Data to send"=""} ("Axis Message")) -> ()  [unwired: 3 in, 1 out]
                n228 = property on="History :" class="LstBox (strict)"("Item Names"=w404) -> ()  [unwired: 2 in, 2 out]
              }
              event "Find index": Value Change {
                n229 = event-data() -> ()  [unwired: 7 out]
                n230 = Format Date/Time String(time format string (%c)="> %H:%M:%S%.3u") -> (date/time string=w421:string)  [unwired: 2 out]
                n231 = property on="History :" class="LstBox (strict)"() -> ("Item Names"=w418:string[])  [unwired: 2 in, 2 out]
                n232 = Concatenate Strings(w421, "  :  " ("string"), "GUI : Find index" ("string")) -> (w420:string)
                n233 = Build Array (concatenate)(w420, w418) -> (w419:string[])
                n234 = Array Subset(array=w419, length=1000) -> (w417:string[])  [unwired: 1 in]
                n235 = property on="History :" class="LstBox (strict)"("Item Names"=w417) -> ()  [unwired: 2 in, 2 out]
                n236 = call "Xeryon Axis SendCommand.vi"("Feedback?"=FALSE, "Stage"=w410, "Axis Command"=T6 {"Command"=enum."Find index", "Data to send"=""} ("Axis Message")) -> ()  [unwired: 3 in, 1 out]
              }
              event "Stop": Value Change {
                n237 = event-data() -> ()  [unwired: 7 out]
                n238 = Format Date/Time String(time format string (%c)="> %H:%M:%S%.3u") -> (date/time string=w434:string)  [unwired: 2 out]
                n239 = property on="History :" class="LstBox (strict)"() -> ("Item Names"=w431:string[])  [unwired: 2 in, 2 out]
                n240 = Concatenate Strings(w434, "  :  " ("string"), "GUI : Stop" ("string")) -> (w433:string)
                n241 = Build Array (concatenate)(w433, w431) -> (w432:string[])
                n242 = Array Subset(array=w432, length=1000) -> (w430:string[])  [unwired: 1 in]
                n243 = property on="History :" class="LstBox (strict)"("Item Names"=w430) -> ()  [unwired: 2 in, 2 out]
                n244 = call "Xeryon Axis SendCommand.vi"("Feedback?"=FALSE, "Stage"=w423, "Axis Command"=T6 {"Command"=enum."Stop", "Data to send"=""} ("Axis Message")) -> ()  [unwired: 3 in, 1 out]
              }
              event "Continue": Value Change {
                n245 = event-data() -> ()  [unwired: 7 out]
                n246 = Format Date/Time String(time format string (%c)="> %H:%M:%S%.3u") -> (date/time string=w447:string)  [unwired: 2 out]
                n247 = property on="History :" class="LstBox (strict)"() -> ("Item Names"=w444:string[])  [unwired: 2 in, 2 out]
                n248 = Concatenate Strings(w447, "  :  " ("string"), "GUI : Continue" ("string")) -> (w446:string)
                n249 = Build Array (concatenate)(w446, w444) -> (w445:string[])
                n250 = Array Subset(array=w445, length=1000) -> (w443:string[])  [unwired: 1 in]
                n251 = property on="History :" class="LstBox (strict)"("Item Names"=w443) -> ()  [unwired: 2 in, 2 out]
                n252 = call "Xeryon Axis SendCommand.vi"("Feedback?"=FALSE, "Stage"=w436, "Axis Command"=T6 {"Command"=enum."Continue", "Data to send"=""} ("Axis Message")) -> ()  [unwired: 3 in, 1 out]
              }
              event "Step -X": Value Change {
                n253 = event-data() -> ()  [unwired: 7 out]
                n254 = Format Date/Time String(time format string (%c)="> %H:%M:%S%.3u") -> (date/time string=w460:string)  [unwired: 2 out]
                n255 = property on="History :" class="LstBox (strict)"() -> ("Item Names"=w457:string[])  [unwired: 2 in, 2 out]
                n256 = Concatenate Strings(w460, "  :  " ("string"), "GUI : Step -X" ("string")) -> (w459:string)
                n257 = Build Array (concatenate)(w459, w457) -> (w458:string[])
                n258 = Array Subset(array=w458, length=1000) -> (w456:string[])  [unwired: 1 in]
                n259 = property on="History :" class="LstBox (strict)"("Item Names"=w456) -> ()  [unwired: 2 in, 2 out]
                n260 = call "Xeryon Axis SendCommand.vi"("Feedback?"=FALSE, "Stage"=w450, "Axis Command"=T6 {"Command"=enum."Step -X", "Data to send"=""} ("Axis Message")) -> ()  [unwired: 3 in, 1 out]
              }
              event "Step +X": Value Change {
                n261 = event-data() -> ()  [unwired: 7 out]
                n262 = Format Date/Time String(time format string (%c)="> %H:%M:%S%.3u") -> (date/time string=w473:string)  [unwired: 2 out]
                n263 = property on="History :" class="LstBox (strict)"() -> ("Item Names"=w470:string[])  [unwired: 2 in, 2 out]
                n264 = Concatenate Strings(w473, "  :  " ("string"), "GUI : Step -X" ("string")) -> (w472:string)
                n265 = Build Array (concatenate)(w472, w470) -> (w471:string[])
                n266 = Array Subset(array=w471, length=1000) -> (w469:string[])  [unwired: 1 in]
                n267 = property on="History :" class="LstBox (strict)"("Item Names"=w469) -> ()  [unwired: 2 in, 2 out]
                n268 = call "Xeryon Axis SendCommand.vi"("Feedback?"=FALSE, "Stage"=w462, "Axis Command"=T6 {"Command"=enum."Step +X", "Data to send"=""} ("Axis Message")) -> ()  [unwired: 3 in, 1 out]
              }
              event "Go": Value Change {
                n269 = event-data() -> ()  [unwired: 7 out]
                n270 = Format Into String(format string="Target position : %d" ("string"), "Desired position") -> (resulting string=w476:string)  [unwired: 2 in, 1 out]
                n271 = Format Date/Time String(time format string (%c)="> %H:%M:%S%.3u") -> (date/time string=w490:string)  [unwired: 2 out]
                n272 = property on="History :" class="LstBox (strict)"() -> ("Item Names"=w487:string[])  [unwired: 2 in, 2 out]
                n273 = Flatten To String(anything="Desired position") -> (data string=w480:string)  [unwired: 3 in, 2 out]
                n274 = Concatenate Strings(w490, "  :  " ("string"), w476) -> (w489:string)
                n275 = Bundle By Name(cluster=T6 {"Command"=enum."Set DPOS", "Data to send"=""} ("Axis Message"), "Data to send"=w480) -> (w479:T6)
                n276 = Build Array (concatenate)(w489, w487) -> (w488:string[])
                n277 = Array Subset(array=w488, length=1000) -> (w486:string[])  [unwired: 1 in]
                n278 = property on="History :" class="LstBox (strict)"("Item Names"=w486) -> ()  [unwired: 2 in, 2 out]
                n279 = call "Xeryon Axis SendCommand.vi"("Feedback?"=FALSE, "Stage"=w478, "Axis Command"=w479) -> ()  [unwired: 3 in, 1 out]
                "Latched setpoint" <- "Desired position"
              }
              event "Apply settings file": Value Change {
                n280 = event-data() -> ()  [unwired: 7 out]
                n281 = Flatten To String(anything="Settings file") -> (data string=w495:string)  [unwired: 3 in, 2 out]
                n282 = Format Date/Time String(time format string (%c)="> %H:%M:%S%.3u") -> (date/time string=w507:string)  [unwired: 2 out]
                n283 = property on="History :" class="LstBox (strict)"() -> ("Item Names"=w504:string[])  [unwired: 2 in, 2 out]
                n284 = Bundle By Name(cluster=T6 {"Command"=enum."Apply settings file", "Data to send"=""} ("Axis Message"), "Data to send"=w495) -> (w494:T6)
                n285 = Concatenate Strings(w507, "  :  " ("string"), "GUI : Apply file" ("string")) -> (w506:string)
                n286 = Build Array (concatenate)(w506, w504) -> (w505:string[])
                n287 = Array Subset(array=w505, length=1000) -> (w503:string[])  [unwired: 1 in]
                n288 = call "Xeryon Axis SendCommand.vi"("Feedback?"=FALSE, "Stage"=w493, "Axis Command"=w494) -> ()  [unwired: 3 in, 1 out]
                n289 = property on="History :" class="LstBox (strict)"("Item Names"=w503) -> ()  [unwired: 2 in, 2 out]
              }
              event "Desired speed": Value Change {
                n290 = event-data() -> ()  [unwired: 7 out]
                n291 = Format Into String(format string="Target speed : %d" ("string"), "Desired speed") -> (resulting string=w509:string)  [unwired: 2 in, 1 out]
                n292 = Format Date/Time String(time format string (%c)="> %H:%M:%S%.3u") -> (date/time string=w523:string)  [unwired: 2 out]
                n293 = property on="History :" class="LstBox (strict)"() -> ("Item Names"=w520:string[])  [unwired: 2 in, 2 out]
                n294 = Flatten To String(anything="Desired speed") -> (data string=w513:string)  [unwired: 3 in, 2 out]
                n295 = Concatenate Strings(w523, "  :  " ("string"), w509) -> (w522:string)
                n296 = Bundle By Name(cluster=T6 {"Command"=enum."Desired speed", "Data to send"=""} ("Axis Message"), "Data to send"=w513) -> (w512:T6)
                n297 = Build Array (concatenate)(w522, w520) -> (w521:string[])
                n298 = Array Subset(array=w521, length=1000) -> (w519:string[])  [unwired: 1 in]
                n299 = property on="History :" class="LstBox (strict)"("Item Names"=w519) -> ()  [unwired: 2 in, 2 out]
                n300 = call "Xeryon Axis SendCommand.vi"("Feedback?"=FALSE, "Stage"=w511, "Axis Command"=w512) -> ()  [unwired: 3 in, 1 out]
              }
              event "Scan -X": Value Change {
                n301 = event-data() -> ("NewVal"=w526:bool)  [unwired: 6 out]
                n302 = Select(t="GUI : Scan -X" ("string"), s=w526, f="GUI : Scan Stop" ("string")) -> (s? t:f=w525:string)
                n303 = Format Date/Time String(time format string (%c)="> %H:%M:%S%.3u") -> (date/time string=w539:string)  [unwired: 2 out]
                n304 = property on="History :" class="LstBox (strict)"() -> ("Item Names"=w536:string[])  [unwired: 2 in, 2 out]
                n305 = Concatenate Strings(w539, "  :  " ("string"), w525) -> (w538:string)
                n306 = case shown="False" w526 {
                  tunnel: [T6 {"Command"=enum."Scan -X", "Data to send"=""} ("Axis Message") T6 {"Command"=enum."Scan Stop", "Data to send"=""} ("Axis Message")] -> w529
                  frame True {
                  }
                  frame False {
                  }
                }
                n307 = Build Array (concatenate)(w538, w536) -> (w537:string[])
                n308 = Array Subset(array=w537, length=1000) -> (w535:string[])  [unwired: 1 in]
                n309 = property on="History :" class="LstBox (strict)"("Item Names"=w535) -> ()  [unwired: 2 in, 2 out]
                n310 = call "Xeryon Axis SendCommand.vi"("Feedback?"=FALSE, "Stage"=w530, "Axis Command"=w529) -> ()  [unwired: 3 in, 1 out]
              }
              event "Scan +X": Value Change {
                n311 = event-data() -> ("NewVal"=w545:bool)  [unwired: 6 out]
                n312 = Select(t="GUI : Scan +X" ("string"), s=w545, f="GUI : Scan Stop" ("string")) -> (s? t:f=w544:string)
                n313 = Format Date/Time String(time format string (%c)="> %H:%M:%S%.3u") -> (date/time string=w557:string)  [unwired: 2 out]
                n314 = property on="History :" class="LstBox (strict)"() -> ("Item Names"=w554:string[])  [unwired: 2 in, 2 out]
                n315 = Concatenate Strings(w557, "  :  " ("string"), w544) -> (w556:string)
                n316 = case shown="True" w545 {
                  tunnel: [T6 {"Command"=enum."Scan +X", "Data to send"=""} ("Axis Message") T6 {"Command"=enum."Scan Stop", "Data to send"=""} ("Axis Message")] -> w548
                  frame True {
                  }
                  frame False {
                  }
                }
                n317 = Build Array (concatenate)(w556, w554) -> (w555:string[])
                n318 = Array Subset(array=w555, length=1000) -> (w553:string[])  [unwired: 1 in]
                n319 = property on="History :" class="LstBox (strict)"("Item Names"=w553) -> ()  [unwired: 2 in, 2 out]
                n320 = call "Xeryon Axis SendCommand.vi"("Feedback?"=FALSE, "Stage"=w543, "Axis Command"=w548) -> ()  [unwired: 3 in, 1 out]
              }
            }
          }
        }
      }
      frame 2 {
        w570 = 0.1 ("y")
        # "Live visualisation of status"
        n321 = call "Xeryon serial data buffer.vi"("Mode"=T7."Get", "Select drive letter"=w572) -> ("Statusbits out"=w563:T3, "Stage data"=w589:T10)  [unwired: 7 in, 5 out]
        "Statusbits" <- w563
        n322 = Unbundle By Name(w589) -> ("Stage type"=→"Stage type":string, "Values out"=w576:i32[], "Parameters out"=w577:T8[])
        n323 = Search 1D Array(1D array=w577, element=Serial_parameters."Encoder position" ("Select parameter")) -> (index of element=w588:i32)  [unwired: 1 in]
        n324 = Search 1D Array(1D array=w577, element=Serial_parameters."Serial number" ("Select parameter")) -> (index of element=w585:i32)  [unwired: 1 in]
        n325 = Search 1D Array(1D array=w577, element=Serial_parameters."Software number" ("Select parameter")) -> (index of element=w582:i32)  [unwired: 1 in]
        n326 = Index Array(array=w576, index=w588) -> (element=w586:i32)
        n327 = Index Array(array=w576, index=w585) -> (element=→"Serial number":i32)
        n328 = Index Array(array=w576, index=w582) -> (element=→"Software number":i32)
        n329 = for {
          tunnel: w577 -> [w601] mode=indexing
          tunnel: w576 -> [w600] mode=indexing
          tunnel: [w597] -> w578 mode=indexing
          n330 = Format Into String(w601) -> (resulting string=w599:string)  [unwired: 3 in, 1 out]
          n331 = Number To Decimal String(number=w600) -> (decimal integer string=w598:string)  [unwired: 1 in]
          n332 = Build Array(w599, w598) -> (w597:string[])
        }
        n333 = call "Xeryon unit conversion.vi"("Type"=w575, "Value in"=w586, "Mode"=T5."Position : To user units") -> ("Value out"=w566:dbl)  [unwired: 2 in]
        "Actual position" <- w566
        n334 = property on="Multicolumn Listbox" class="MCListbox (strict)"("ItemNames"=w578) -> ()  [unwired: 2 in, 2 out]
        n335 = local read "Desired position"() -> (w571:dbl)
        n336 = Unbundle By Name(w563) -> ("Position reached"=w562:bool)
        n337 = local read "Latched setpoint"() -> (w565:dbl)
        n338 = Add(x=w571, y=w570) -> (x+y=w569:dbl)
        n339 = Subtract(x=w571, y=w570) -> (x-y=w568:dbl)
        n340 = In Range and Coerce(upper limit=w569, x=w566, lower limit=w568) -> (In Range?=w567:bool)  [unwired: 1 out]
        "Within Tolerance" <- w567
        n341 = Boolean To (0,1)(Boolean=w562) -> (0, 1=w561:i16)
        n342 = Bundle("Value out"=w566, "Latched setpoint"=w565, w561) -> (→"Waveform Chart":T4)  [unwired: 1 in]
        n343 = call "Xeryon serial data buffer.vi"("Mode"=T7."Update position", "Position in"=w566, "Within tol in"=w567, "Select drive letter"=w572) -> ()  [unwired: 5 in, 7 out]
        n344 = Select(t=98, s=w591, f=3 ("t")) -> (s? t:f=w592:i32)
      }
      frame 3 {
        # "Enable/disable buttons"
        n345 = local read "Statusbits"() -> (w604:T3)
        n346 = Unbundle By Name(w604) -> ("Motor On"=w614:bool)
        n347 = Unbundle By Name(w604) -> ("Motor On"=w612:bool, "Scanning"=w611:bool)
        n348 = Compound Arithmetic op=AND(w612, invert w611) -> (w610:bool)
        n349 = Select(t=2, s=w614, f=0) -> (s? t:f=w613:i32)
        n350 = Select(t=2, s=w610, f=0) -> (s? t:f=w609:i32)
        n351 = property on="Find index" class="Bool"("DisabledEnum"=w613) -> ()  [unwired: 2 in, 2 out]
        n352 = property on="Continue" class="Bool"("DisabledEnum"=w613) -> ()  [unwired: 2 in, 2 out]
        n353 = property on="Step -X" class="Bool"("DisabledEnum"=w613) -> ()  [unwired: 2 in, 2 out]
        n354 = property on="Go" class="Bool"("DisabledEnum"=w613) -> ()  [unwired: 2 in, 2 out]
        n355 = property on="Step +X" class="Bool"("DisabledEnum"=w613) -> ()  [unwired: 2 in, 2 out]
        n356 = property on="Scan -X" class="Bool (strict)"("DisabledEnum"=w609) -> ()  [unwired: 2 in, 2 out]
        n357 = property on="Scan +X" class="Bool (strict)"("DisabledEnum"=w609) -> ()  [unwired: 2 in, 2 out]
      }
      frame 98 {
        w619 = T11 0 items=["no dialog", "OK message", "continue or stop message", "OK message + warnings", "continue/stop + warnings"] ("type of dialog (OK msg:1)")
        # "Error handler"
        n358 = call <vilib>:"Simple Error Handler.vi"("type of dialog (OK msg:1)"=w619, "error in (no error)"=w620) -> ("message"=w618:string)  [unwired: 3 in, 4 out]
        n359 = Format Into String(format string="An error occured with the Xeryon serial communication.\n\n%s" ("Algemene omschrijving"), w618) -> (resulting string=w617:string)  [unwired: 2 in, 1 out]
        n360 = Format Date/Time String(time format string (%c)="> %H:%M:%S%.3u") -> (date/time string=w626:string)  [unwired: 2 out]
        n361 = Concatenate Strings("Error message : " ("string"), w618) -> (w622:string)
        n362 = One Button Dialog(message=w617) -> ()  [unwired: 1 in, 1 out]
        n363 = property on="History :" class="LstBox (strict)"() -> ("Item Names"=w631:string[])  [unwired: 2 in, 2 out]
        n364 = Concatenate Strings(w626, "  :  " ("string"), w622) -> (w628:string)
        n365 = Build Array (concatenate)(w628, w631) -> (w629:string[])
        n366 = Array Subset(array=w629, length=1000) -> (w624:string[])  [unwired: 1 in]
        n367 = property on="History :" class="LstBox (strict)"("Item Names"=w624) -> ()  [unwired: 2 in, 2 out]
      }
      frame 99 {
        # "Exit"
        n368 = Release Queue(queue=w636) -> ()  [unwired: 1 in, 4 out]
      }
    }
  }
  n369 = disable-structure shown="Disabled" {
    frame Disabled {
      n370 = call "Xeryon Axis SendCommand.vi"() -> ()  [unwired: 6 in, 1 out]
      n371 = call "Xeryon SetDPos command.vi"() -> ()  [unwired: 6 in]
    }
    frame Enabled {
    }
  }
